vi "robotics_state.vi"() -> (0 "error out":errorcluster, 3 "Notifier out":refnum<notifier>)   [LabVIEW 2013]
uses:
  main_machine/type_defs/robotics_states.ctl
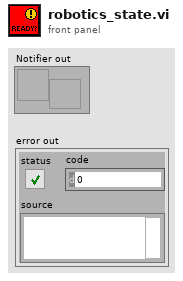
[diagram p1: front panel]
types:
  T1 = typedef "robotics_states.ctl" = enum16{"BUSY", "READY"}
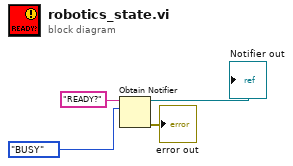
[diagram p0: block diagram]
diagram:
  n1 = Obtain Notifier(name (unnamed)="READY?", notification data type=robotics_states."BUSY") -> (notifier out=→"Notifier out":refnum<notifier>, error out=→"error out":errorcluster)  [unwired: 2 in, 1 out]
